vi "get contained vis.vi"(8 "error in":errorcluster, 11 "ProjectItem in":refnum<vi>) -> (0 "error out":errorcluster, 1 "ids":string[](array[string]), 2 "paths":path[](array[path]), 3 "ProjectItem out":refnum<vi>)   [LabVIEW 2013]
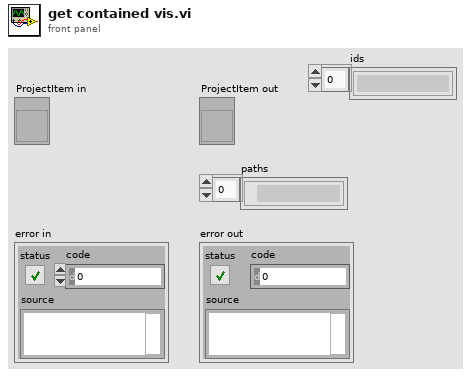
[diagram p1: front panel]
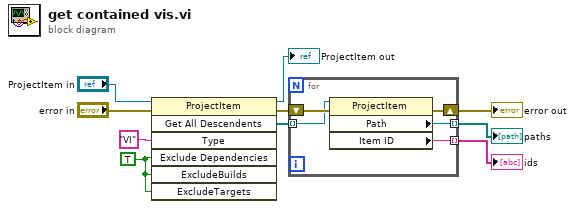
[diagram p0: block diagram]
diagram:
  w2 = TRUE ("ExcludeTargets")
  n1 = invoke class="ProjectItem" method="Get All Descendents"(reference="ProjectItem in", error in="error in", "Type"="VI", "Exclude Dependencies"=w2, "ExcludeBuilds"=w2, "ExcludeTargets"=w2) -> (reference out=→"ProjectItem out":refnum<vi>, error out=w7:errorcluster, "All Descendents"=w3:refnum<vi>[])  [unwired: 1 in, 4 out]
  n2 = for {
    tunnel: [w14] -> w9 mode=indexing
    shift-right: [w13] -> w10
    shift-left: w7 -> [w12]
    tunnel: w3 -> [w11] mode=indexing
    tunnel: [w15] -> w1 mode=indexing
    n3 = property class="ProjectItem"(reference=w11, error in=w12) -> (error out=w13:errorcluster, "Path"=w14:path, "Item ID"=w15:string)  [unwired: 1 out]
  }
  "error out" <- w10
  "paths" <- w9
  "ids" <- w1
